vi "FGUDP.vi"(5 "Remote Port":u16=5502, 7 "Remote Host":string="10.0.22.163", 8 "Error In":errorcluster, 10 "Data String":string, 11 "UDP State":T1) -> (0 "error out":errorcluster)   [LabVIEW 2010, in "Flight Gear Interface Custom Device.lvlib"]
uses:
  Flight Gear Interface Custom Device.lvlib
  FlightGearState.ctl
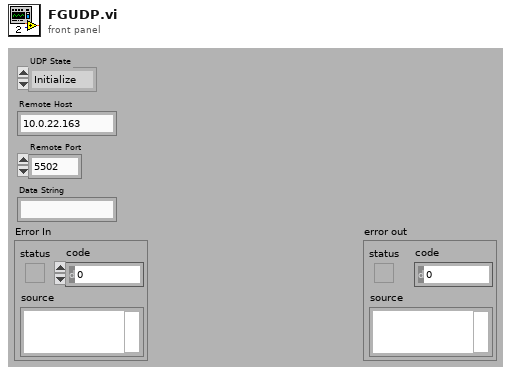
[diagram p1: front panel]
types:
  T1 = typedef "Flight Gear Interface Custom Device.lvlib/FlightGearState.ctl" = enum16{"Initialize", "Write", "Close"}
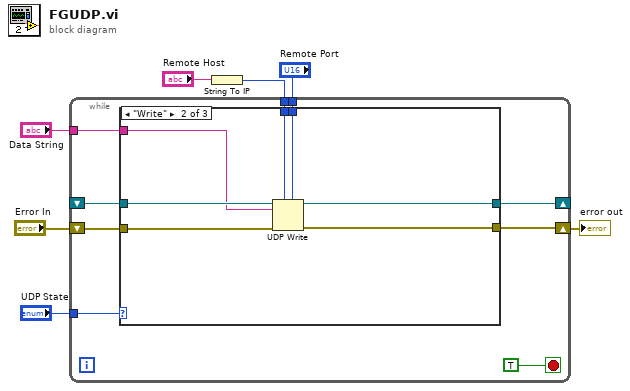
[diagram p0: block diagram]
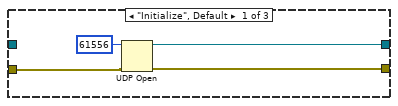
[diagram p2: hidden frame]
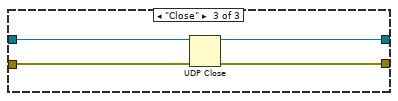
[diagram p3: hidden frame]
diagram:
  n1 = String To IP(1:"Remote Host") -> (0:w3:u32)
  n2 = while {
    tunnel: "UDP State" -> [w16]
    shift-right: [w14] -> w2
    shift-left: "Error In" -> [w15]
    shift-right: [w12] -> _
    shift-left: _ -> [w11]
    tunnel: "Remote Port" -> [w10]
    tunnel: w3 -> [w9]
    tunnel: "Data String" -> [w8]
    stop <- TRUE stop-if-true
    n3 = case shown="\"Write\"" w16 {
      tunnel: w15 -> [w19 w25 w28]
      tunnel: [w18 w24 w29] -> w14
      tunnel: [w17 w26 w30] -> w12
      tunnel: w11 -> [_ w27 w31]
      tunnel: w10 -> [_ w23 _]
      tunnel: w9 -> [_ w22 _]
      tunnel: w8 -> [_ w21 _]
      frame "Initialize", Default {
        n4 = UDP Open(8:w19, 11:u16 61556 ("port")) -> (port=w17:refnum<k16>, 0:w18:errorcluster)  [unwired: 3 in, 1 out]
      }
      frame "Write" {
        n5 = UDP Write(address=w22, port or service name=w23, connection ID=w27, data in=w21, 8:w25) -> (error out=w24:errorcluster, 3:w26:refnum<k16>)  [unwired: 1 in]
      }
      frame "Close" {
        n6 = UDP Close(connection ID=w31, 8:w28) -> (connection ID out=w30:refnum<k16>, error out=w29:errorcluster)
      }
    }
  }
  "error out" <- w2
